vi "Get VI Refs and Info.vi"(8 "error in (no error)":errorcluster, 11 "Path to analyze":path) -> (0 "error out":errorcluster, 1 "output cluster":T1, 2 "Name":string, 3 "VI out":refnum<vi>)   [LabVIEW 2018, in "Name and Dependency Processing.lvlib"]
uses:
  Name and Dependency Processing.lvlib
  Dep Names and Paths.ctl
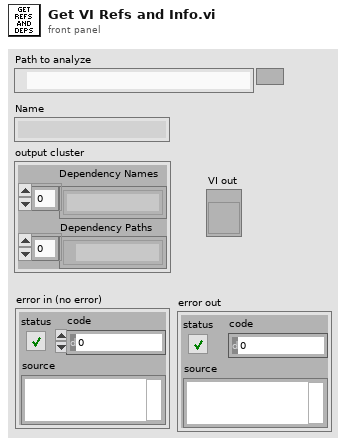
[diagram p1: front panel]
types:
  T1 = typedef "Name and Dependency Processing.lvlib/Dep Names and Paths.ctl" = cluster{"Dependency Names":string[], "Dependency Paths":path[]}
  T2 = enum8{"Include the clone VI", "Include the original reentrant VI instead of the clone VI", "Include both the original reentrant VI and the clone VI"}
  T3 = enum8{"No dynamic dispatch VIs", "Include nearest implementation", "Include all overrides"}
  T4 = enum8{"Only include commented out diagrams if diagram already loaded", "Never include commented out diagrams", "Always include commented out diagrams"}
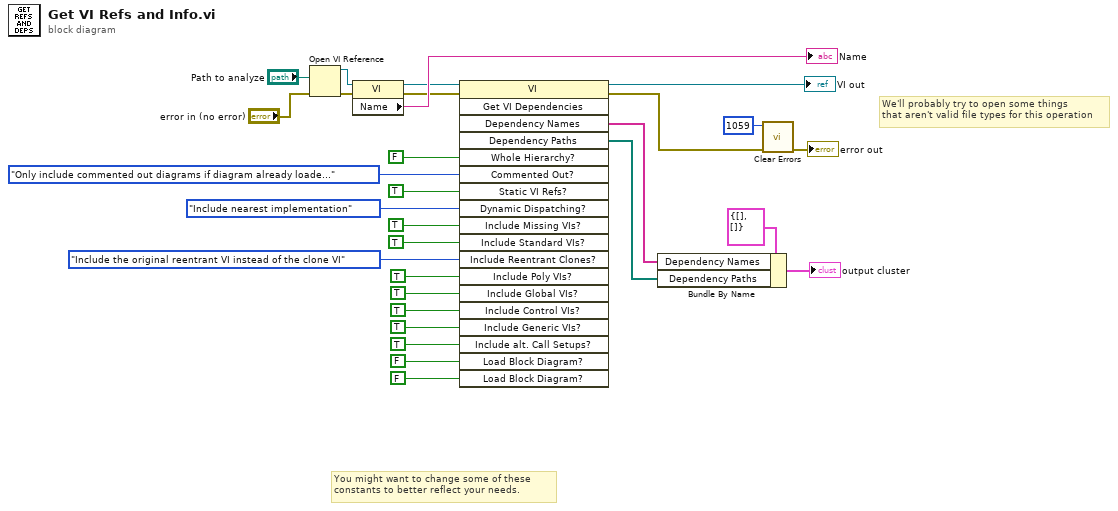
[diagram p0: block diagram]
diagram:
  # "We'll probably try to open some things \nthat aren't valid file types for this operation"
  # "You might want to change some of these \nconstants to better reflect your needs."
  n1 = Open VI Reference(vi path="Path to analyze", error in (no error)="error in (no error)") -> (vi reference=w25:refnum<vi>, error out=w9:errorcluster)  [unwired: 4 in]
  n2 = property class="VI"(reference=w25, error in=w9) -> (reference out=w26:refnum<vi>, error out=w24:errorcluster, "Name"=→"Name":string)
  n3 = invoke class="VI" method="Get VI Dependencies"(reference=w26, error in=w24, "Whole Hierarchy?"=FALSE, "Commented Out?"=T4."Only include commented out diagrams if diagram already loaded" ("Commented Out Diagrams?"), "Static VI Refs?"=TRUE, "Dynamic Dispatching?"=T3."Include nearest implementation", "Include Missing VIs?"=TRUE ("Include Missing Items?"), "Include Standard VIs?"=TRUE, "Include Reentrant Clones?"=T2."Include the original reentrant VI instead of the clone VI", "Include Poly VIs?"=TRUE, "Include Global VIs?"=TRUE, "Include Control VIs?"=TRUE, "Include Generic VIs?"=TRUE, "Include alt. Call Setups?"=TRUE ("Include Alternate Call Setups?"), "Load Block Diagram?"=FALSE ("Keep Express and Malleable VIs?"), "Load Block Diagram?"=FALSE) -> (reference out=→"VI out":refnum<vi>, error out=w3:errorcluster, "Dependency Names"=w6:string[], "Dependency Paths"=w5:path[])  [unwired: 3 in, 15 out]
  n4 = Bundle By Name(cluster=T1 {"Dependency Names"=[], "Dependency Paths"=[]} ("Dependencies 2"), "Dependency Names"=w6, "Dependency Paths"=w5) -> (→"output cluster":T1)
  n5 = call <vilib>:"Clear Errors.vi"("error in (no error)"=w3, "specific error code to clear (0: all)"=1059) -> ("error out"=→"error out":errorcluster)  [unwired: 4 in, 1 out]
